vi "Choose_best_target.vi"(0 "R1mag lower limit":dbl, 2 "FOV":dbl, 3 "Footprint":dbl, 5 "PM limit":dbl, 6 "EPOCH TEL":dbl format="%.3f", 8 "DEC TEL":dbl format="%<%H:%M:%S>t", 9 "Table Astrometry":T1 {"CRVAL" format="%.6g"; "CD" format="%_8g"; "NAXIS" format="%#.0f"}, 10 "RA TEL":dbl format="%<%H:%M:%S%1u>t", 12 "USNO_data":string[][](array[string])) -> (13 "erreur":bool, 14 "target RA":dbl format="%<%H:%M:%S%2u>t", 15 "target DEC":dbl format="%<%H:%M:%S%1u>t", 16 "target EPOCH":dbl format="%.3f", 17 "target R1mag":dbl format="%.2f", 18 "target RA (deg)":dbl format="%#.6f", 19 "target DEC (deg)":dbl format="%#.6f")   [LabVIEW 2011]
panel:
  out "R-I":dbl
  out "B-R":dbl
  out "target X":dbl
  out "target Y":dbl
  out "Data OUT":string[][](array[string])
  out "Best Target":string[](array[string])
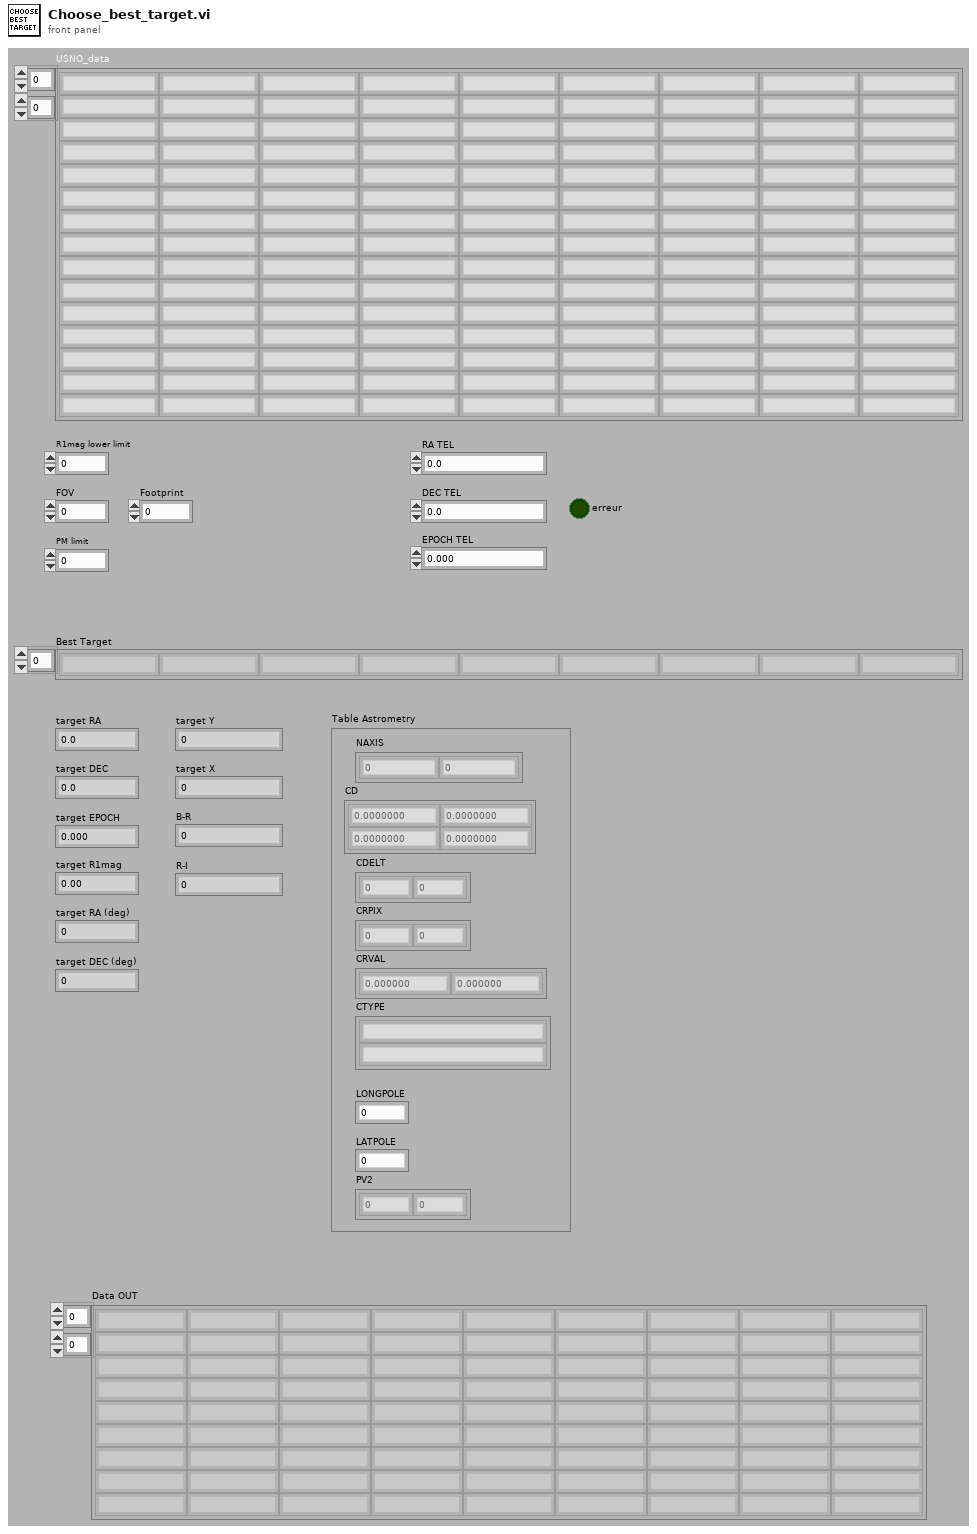
[diagram p1: front panel]
types:
  T1 = cluster{"NAXIS":dbl[], "CD":dbl[][], "CDELT":dbl[], "CRPIX":dbl[], "CTYPE":string[], "CRVAL":dbl[], "LONGPOLE":dbl, "LATPOLE":dbl, "PV2":dbl[]}
  T2 = cluster{"crit":string, "String":string, "String":string, "String":string, "String":string, "String":string, "String":string, "String":string, "String":string}[]
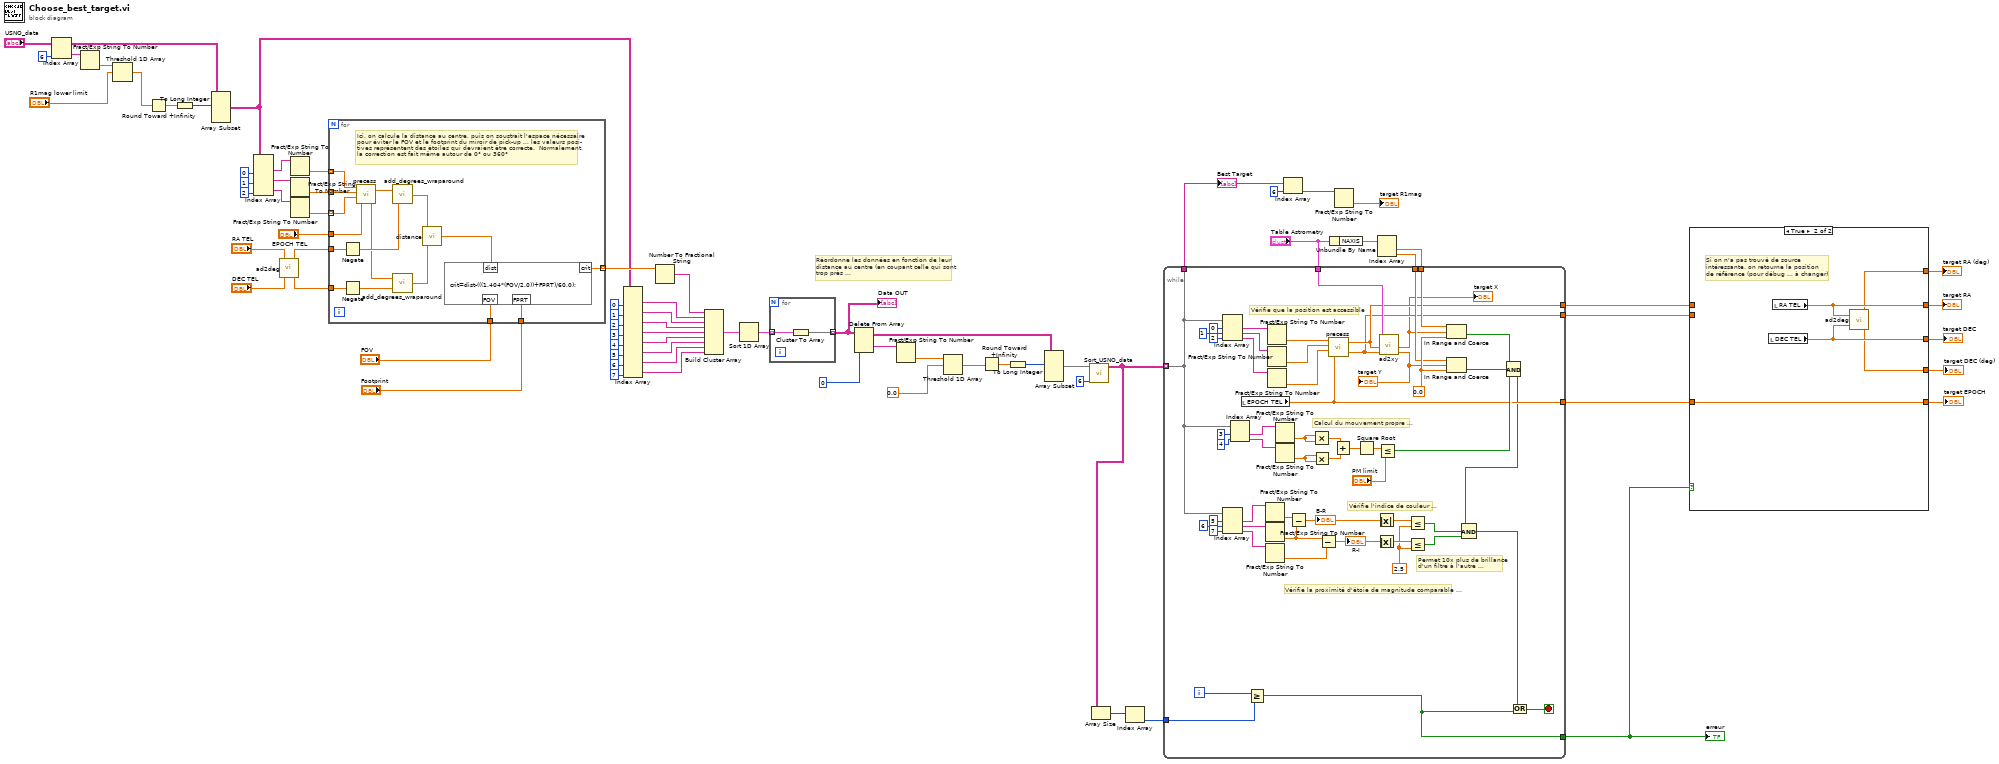
[diagram p0: block diagram]
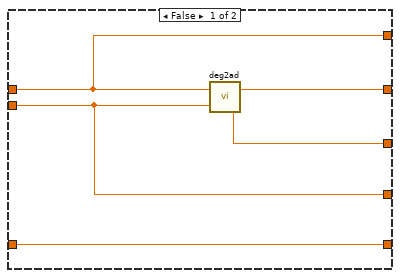
[diagram p2: hidden frame]
diagram:
  # "Réordonne les données en fonction de leur\ndistance au centre (en coupant celle qui sont\ntrop près ..."
  n1 = Index Array(array="USNO_data", index (col)=6 ("disabled index (col)")) -> (element=w75:string[])  [unwired: 1 in]
  n2 = Fract/Exp String To Number(string=w75) -> (number=w74:dbl[])  [unwired: 3 in, 1 out]
  n3 = Threshold 1D Array(2:"R1mag lower limit", 3:w74) -> (0:w72:dbl)  [unwired: 1 in]
  n4 = Round Toward +Infinity(x=w72) -> (ceil(x): smallest int >= x=w71:dbl)
  n5 = To Long Integer(number=w71) -> (32bit integer=w70:i32)
  n6 = Array Subset(array="USNO_data", index (row)=w70) -> (w34:string[][])  [unwired: 3 in]
  n7 = Index Array(array=w34, index (col) #1=0 ("disabled index (col)"), index (col) #2=1 ("index (col)"), index (col) #3=2 ("index (col)")) -> (element #1=w66:string[], element #2=w65:string[], element #3=w64:string[])  [unwired: 3 in]
  n8 = call "ad2deg.vi"("DEC (sec)"="DEC TEL", "RA (sec)"="RA TEL") -> ("DEC (°)"=w56:dbl, "RA (°)"=w58:dbl)
  n9 = Fract/Exp String To Number(string=w66) -> (number=w63:dbl[])  [unwired: 3 in, 1 out]
  n10 = Fract/Exp String To Number(string=w65) -> (number=w62:dbl[])  [unwired: 3 in, 1 out]
  n11 = Fract/Exp String To Number(string=w64) -> (number=w61:dbl[])  [unwired: 3 in, 1 out]
  n12 = for {
    tunnel: w63 -> [w92] mode=indexing
    tunnel: w62 -> [w91] mode=indexing
    tunnel: w61 -> [w90] mode=indexing
    tunnel: "EPOCH TEL" -> [w89]
    tunnel: w58 -> [w88]
    tunnel: w56 -> [w87]
    tunnel: "FOV" -> [w79]
    tunnel: "Footprint" -> [w80]
    tunnel: [w77] -> w35 mode=indexing
    # "Ici, on calcule la distance au centre, puis on soustrait l'espace nécessaire\npour éviter le FOV et le footprint du miroir de pick-up ... les valeurs posi-\ntives représentent des étoiles qui devraient être correcte.  Normalement,\nla correction est fait même autour de 0° ou 360°"
    n13 = Negate(x=w88) -> (-x=w85:dbl)
    n14 = Negate(x=w87) -> (-x=w84:dbl)
    n15 = call "precess.vi"("Eq2"=w89, "Eq1"=w90, "DEC 1"=w91, "RA 1"=w92) -> ("DEC 2"=w83:dbl, "RA 2"=w86:dbl)
    n16 = call "add_degrees_wraparound.vi"("DEG 2"=w85, "DEG 1"=w86) -> ("DEG OUT"=w82:dbl)
    n17 = call "add_degrees_wraparound.vi"("DEG 2"=w84, "DEG 1"=w83) -> ("DEG OUT"=w81:dbl)
    n18 = call "distance.vi"("D2"=w81, "D1"=w82) -> ("DT"=w78:dbl)
    n19 = formula code="crit=dist-(((1.404*(FOV/2.0))+FPRT)/60.0);"("FOV"=w79, "FPRT"=w80, "dist"=w78) -> ("crit"=w77:dbl)
  }
  n20 = Index Array(array=w34, index (col) #1=0 ("index (col)"), index (col) #2=1 ("index (col)"), index (col) #3=2 ("index (col)"), index (col) #4=3 ("index (col)"), index (col) #5=4 ("index (col)"), index (col) #6=5 ("index (col)"), index (col) #7=6 ("index (col)"), index (col) #8=7 ("index (col)")) -> (element #1=w44:string[], element #2=w45:string[], element #3=w46:string[], element #4=w47:string[], element #5=w48:string[], element #6=w49:string[], element #7=w50:string[], element #8=w51:string[])  [unwired: 8 in]
  n21 = Number To Fractional String(number=w35) -> (F-format string=w33:string[])  [unwired: 3 in]
  n22 = Build Cluster Array(w33, w44, w45, w46, w47, w48, w49, w50, w51) -> (w52:T2)
  n23 = Sort 1D Array(array=w52) -> (sorted array=w53:T2)
  n24 = for {
    tunnel: w53 -> [w94] mode=indexing
    tunnel: [w93] -> w9 mode=indexing
    n25 = Cluster To Array(cluster=w94) -> (array=w93:string[])
  }
  "Data OUT" <- w9
  n26 = Delete From Array(array=w9, index (col)=0 ("disabled index (col)")) -> (deleted portion=w32:string[], array with subset deleted=w23:string[][])  [unwired: 2 in]
  n27 = Fract/Exp String To Number(string=w32) -> (number=w31:dbl[])  [unwired: 3 in, 1 out]
  n28 = Threshold 1D Array(2:0.0 ("threshold y"), 3:w31) -> (0:w27:dbl)  [unwired: 1 in]
  n29 = Round Toward +Infinity(x=w27) -> (ceil(x): smallest int >= x=w28:dbl)
  n30 = To Long Integer(number=w28) -> (32bit integer=w29:i32)
  n31 = Array Subset(array=w23, index (row)=w29) -> (w26:string[][])  [unwired: 3 in]
  n32 = call "Sort_USNO_data.vi"("Column Used"=6, "Data IN"=w26) -> ("Data OUT"=w8:string[][])  [unwired: 8 in, 1 out]
  n33 = Array Size(array=w8) -> (size(s)=w10:i32[])
  n34 = Index Array(array=w10) -> (element=w7:i32)  [unwired: 1 in]
  n35 = Unbundle By Name("Table Astrometry") -> ("NAXIS"=w21:dbl[])
  n36 = Index Array(array=w21) -> (element #1=w19:dbl, element #2=w18:dbl)  [unwired: 2 in]
  n37 = while {
    tunnel: w8 -> [w111] mode=indexing
    tunnel: "Table Astrometry" -> [w129]
    tunnel: w19 -> [w127]
    tunnel: w18 -> [w126]
    tunnel: [w122] -> w13
    tunnel: [w121] -> w12
    tunnel: [w120] -> w17
    tunnel: [w111] -> w16
    tunnel: w7 -> [w115]
    tunnel: [w114] -> w6
    i -> [w116]
    stop <- w117 stop-if-true
    w99 = 2.5 ("y")
    w128 = 0.0
    # "Vérifie la proximité d'étoie de magnitude comparable ..."
    # "Permet 10x plus de brillance\nd'un filtre à l'autre ..."
    # "Vérifie l'indice de couleur ..."
    # "Vérifie que la position est accessible"
    # "Calcul du mouvement propre ..."
    n38 = Index Array(array=w111, index #1=0 ("index"), index #2=1 ("index"), index #3=2 ("index")) -> (element #1=w133:string, element #2=w132:string, element #3=w135:string)
    n39 = Index Array(array=w111, index #1=5 ("index (row)"), index #2=6 ("index (row)"), index #3=7 ("index")) -> (element #1=w109:string, element #2=w108:string, element #3=w107:string)
    n40 = Index Array(array=w111, index #1=3 ("index (row)"), index #2=4 ("index (row)")) -> (element #1=w143:string, element #2=w144:string)
    n41 = local read "EPOCH TEL"() -> (w120:dbl)
    n42 = Greater Or Equal?(x=w116, y=w115) -> (x >= y?=w114:bool)
    n43 = Fract/Exp String To Number(string=w109) -> (number=w106:dbl)  [unwired: 3 in, 1 out]
    n44 = Fract/Exp String To Number(string=w108) -> (number=w105:dbl)  [unwired: 3 in, 1 out]
    n45 = Fract/Exp String To Number(string=w107) -> (number=w104:dbl)  [unwired: 3 in, 1 out]
    n46 = Fract/Exp String To Number(string=w133) -> (number=w138:dbl)  [unwired: 3 in, 1 out]
    n47 = Fract/Exp String To Number(string=w132) -> (number=w137:dbl)  [unwired: 3 in, 1 out]
    n48 = Fract/Exp String To Number(string=w135) -> (number=w136:dbl)  [unwired: 3 in, 1 out]
    n49 = Fract/Exp String To Number(string=w143) -> (number=w145:dbl)  [unwired: 3 in, 1 out]
    n50 = Fract/Exp String To Number(string=w144) -> (number=w146:dbl)  [unwired: 3 in, 1 out]
    n51 = Subtract(x=w106, y=w105) -> (x-y=w103:dbl)
    "B-R" <- w103
    n52 = Multiply(x=w145, y=w145) -> (x*y=w147:dbl)
    n53 = Multiply(x=w146, y=w146) -> (x*y=w148:dbl)
    n54 = Subtract(x=w105, y=w104) -> (x-y=w102:dbl)
    "R-I" <- w102
    n55 = call "precess.vi"("Eq2"=w120, "Eq1"=w136, "DEC 1"=w137, "RA 1"=w138) -> ("DEC 2"=w121:dbl, "RA 2"=w122:dbl)
    n56 = Add(x=w147, y=w148) -> (x+y=w149:dbl)
    n57 = Square Root(x=w149) -> (sqrt(x)=w140:dbl)
    n58 = Absolute Value(x=w103) -> (abs(x)=w101:dbl)
    n59 = Absolute Value(x=w102) -> (abs(x)=w100:dbl)
    n60 = Less Or Equal?(x=w140, y="PM limit") -> (x <= y?=w125:bool)
    n61 = call "ad2xy.vi"("DEC"=w121, "RA"=w122, "Astrometry"=w129) -> ("Y"=w118:dbl, "X"=w119:dbl)  [unwired: 6 in, 1 out]
    "target Y" <- w118
    "target X" <- w119
    n62 = Less Or Equal?(x=w101, y=w99) -> (x <= y?=w98:bool)
    n63 = Less Or Equal?(x=w100, y=w99) -> (x <= y?=w97:bool)
    n64 = In Range and Coerce(upper limit=w127, x=w119, lower limit=w128) -> (In Range?=w124:bool)  [unwired: 1 out]
    n65 = In Range and Coerce(upper limit=w126, x=w118, lower limit=w128) -> (In Range?=w123:bool)  [unwired: 1 out]
    n66 = Compound Arithmetic op=AND(w124, w123, w125) -> (w96:bool)
    n67 = Compound Arithmetic op=AND(w96, w98, w97) -> (w95:bool)
    n68 = Or(x=w95, y=w114) -> (x .or. y?=w117:bool)
  }
  "Best Target" <- w16
  "erreur" <- w6
  n69 = Index Array(array=w16, index=6) -> (element=w14:string)
  n70 = Fract/Exp String To Number(string=w14) -> (number=→"target R1mag":dbl)  [unwired: 3 in, 1 out]
  n71 = case shown="True" w6 {
    tunnel: w17 -> [w150 w155]
    tunnel: w13 -> [w151 _]
    tunnel: w12 -> [w152 _]
    tunnel: [w154 w158] -> w5
    tunnel: [w153 w159] -> w4
    tunnel: [w152 w156] -> w3
    tunnel: [w151 w157] -> w2
    tunnel: [w150 w155] -> w1
    frame False {
      n72 = call "deg2ad.vi"("DEC (°)"=w152, "RA (°)"=w151) -> ("DEC (°)"=w153:dbl, "RA (sec)"=w154:dbl)
    }
    frame True {
      # "Si on n'a pas trouvé de source\nintéressante, on retourne la position\nde référence (pour débug ... à changer)"
      n73 = local read "DEC TEL"() -> (w159:dbl)
      n74 = local read "RA TEL"() -> (w158:dbl)
      n75 = call "ad2deg.vi"("DEC (sec)"=w159, "RA (sec)"=w158) -> ("DEC (°)"=w156:dbl, "RA (°)"=w157:dbl)
    }
  }
  "target RA" <- w5
  "target DEC" <- w4
  "target DEC (deg)" <- w3
  "target RA (deg)" <- w2
  "target EPOCH" <- w1
